vi "get runtime class name.vi"(8 "error in":errorcluster, 11 "sample module configuration in":refnum<class "sample module configuration.lvclass">) -> (0 "error out":errorcluster, 2 "class name":string, 3 "sample module configuration out":refnum<class "sample module configuration.lvclass">)   [LabVIEW 2013, in "sample module configuration.lvclass"]
doc: "Provides an interface for determining the module runtime class associated with this module configuration. This class name can then be used to dynamically load or locate the runtime class for initialization purposes."
uses:
  sample module configuration.lvclass
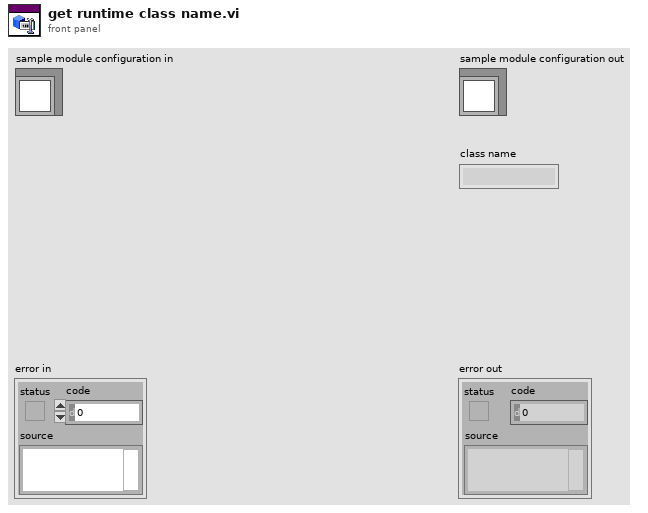
[diagram p1: front panel]
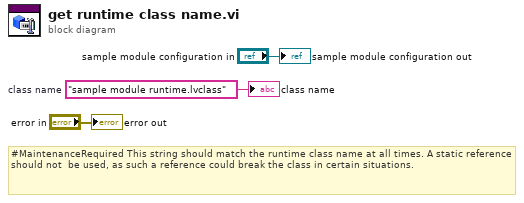
[diagram p0: block diagram]
diagram:
  w1 = "sample module runtime.lvclass"  # class name
  # "#MaintenanceRequired This string should match the runtime class name at all times. A static reference should not  be used, as such a reference could break the class in certain situations."
  "error out" <- "error in"
  "sample module configuration out" <- "sample module configuration in"
  "class name" <- w1
